vi "Microsync demo.vi"() -> ()   [LabVIEW 2023]
uses:
  4b1e20da-cac2-45f8-90a9-c1f199967da0.vi
  34aa4032-f9e1-440a-b4b5-18c951d9b119.vi
  <vilib>/Instr/_visa.llb/VISA Configure Serial Port (Instr).vi
  <vilib>/Instr/_visa.llb/VISA Flush IO Buffer Mask.ctl
panel:
  out "read buffer":string
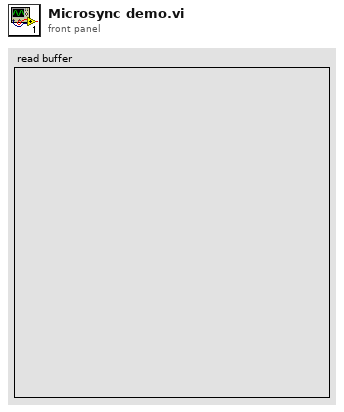
[diagram p1: front panel]
types:
  T1 = typedef "VISA Flush IO Buffer Mask.ctl" = u16
  T2 = cluster{"interval_us":u32, "N":u32, "timestamp_us":u32, "arg2":u32, "arg1":u32}
  T3 = cluster{"interval_us":u32, "N":u32, "timestamp_us":u32, "arg2":u32, "Pin":string}
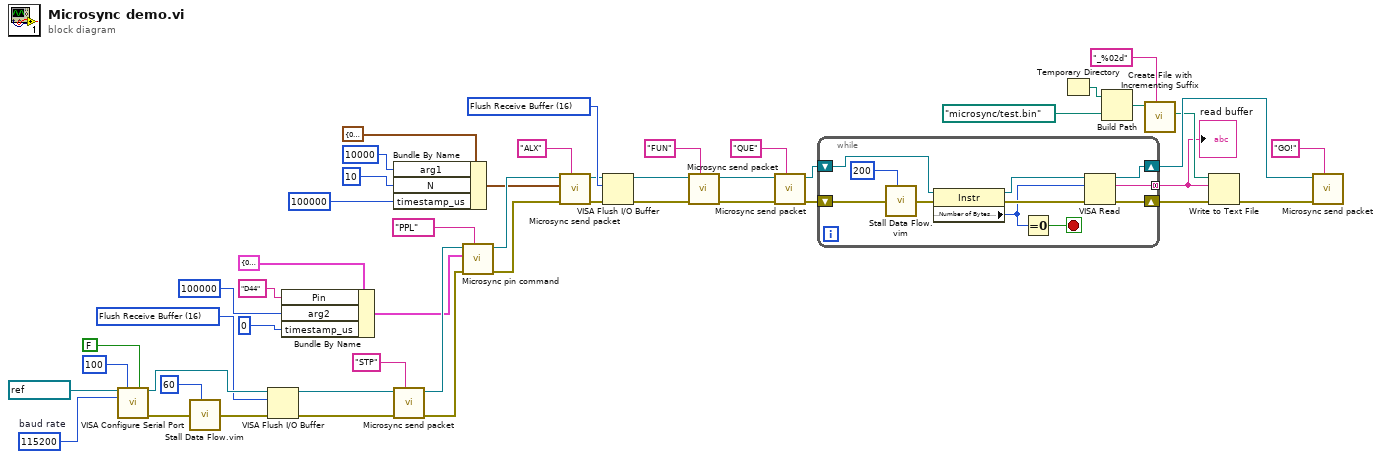
[diagram p0: block diagram]
diagram:
  w5 = T1 16 items=["Flush Receive Buffer"=16, "Write Transmit Buffer to Device"=32, "Flush Receive Buffer (No I/O)"=64, "Flush Transmit Buffer"=128] ("Mask")
  w6 = T1 16 items=["Flush Receive Buffer"=16, "Write Transmit Buffer to Device"=32, "Flush Receive Buffer (No I/O)"=64, "Flush Transmit Buffer"=128] ("Mask")
  w48 = u32 115200  # baud rate
  n1 = call-poly "VISA Configure Serial Port"("VISA resource name"=refnum<visa-resource-name> "COM5", "timeout (10sec)"=u32 100, "Enable Termination\nChar (T)"=FALSE ("Enable Termination\nChar (T)"), "baud rate (9600)"=w48) -> ("VISA resource name out"=w47:refnum<visa-resource-name>, "error out"=w46:errorcluster)  [unwired: 10 in]
  n2 = call "Stall Data Flow.vim"("value in"=w46, "milliseconds to wait"=u32 60) -> ("value out"=w45:errorcluster)  [unwired: 1 out]
  n3 = VISA Flush I/O Buffer(VISA resource name=w47, mask (16)=w6, error in (no error)=w45) -> (VISA resource name out=w34:refnum<visa-resource-name>, error out=w33:errorcluster)
  n4 = Bundle By Name(cluster=T3 {"interval_us"=0, "N"=0, "timestamp_us"=0, "arg2"=0, "Pin"=""} ("Arguments"), "Pin"="D44", "arg2"=u32 100000, "timestamp_us"=u32 0) -> (w36:T3)
  n5 = Bundle By Name(cluster=T2 {"interval_us"=0, "N"=0, "timestamp_us"=0, "arg2"=0, "arg1"=0} ("Arguments"), "arg1"=u32 10000, "N"=u32 10, "timestamp_us"=u32 100000) -> (w28:T2)
  n6 = call "Microsync send packet.vi"("Command"="STP", "error in (no error)"=w33, "VISA resource name"=w34) -> ("error out"=w35:errorcluster, "VISA resource name out"=w41:refnum<visa-resource-name>)  [unwired: 6 in, 1 out]
  n7 = call "Microsync pin command.vi"("Combo Box"="PPL", "error in (no error)"=w35, "Arguments"=w36, "VISA resource name"=w41) -> ("error out"=w24:errorcluster, "VISA resource name out"=w30:refnum<visa-resource-name>)  [unwired: 5 in, 1 out]
  n8 = call "Microsync send packet.vi"("Command"="ALX", "error in (no error)"=w24, "Arguments"=w28, "VISA resource name"=w30) -> ("error out"=w1:errorcluster, "VISA resource name out"=w4:refnum<visa-resource-name>)  [unwired: 5 in, 1 out]
  n9 = VISA Flush I/O Buffer(VISA resource name=w4, mask (16)=w5, error in (no error)=w1) -> (VISA resource name out=w3:refnum<visa-resource-name>, error out=w2:errorcluster)
  n10 = call "Microsync send packet.vi"("Command"="FUN", "error in (no error)"=w2, "VISA resource name"=w3) -> ("error out"=w13:errorcluster, "VISA resource name out"=w14:refnum<visa-resource-name>)  [unwired: 6 in, 1 out]
  n11 = call "Microsync send packet.vi"("Command"="QUE", "error in (no error)"=w13, "VISA resource name"=w14) -> ("error out"=w7:errorcluster, "VISA resource name out"=w10:refnum<visa-resource-name>)  [unwired: 6 in, 1 out]
  n12 = while {
    shift-right: [w51] -> w16
    shift-left: w7 -> [w53]
    shift-right: [w60] -> w19
    shift-left: w10 -> [w58]
    tunnel: [w59] -> w17 mode=concatenating
    stop <- w56 stop-if-true
    n13 = call "Stall Data Flow.vim"("value in"=w53, "milliseconds to wait"=u32 200) -> ("value out"=w52:errorcluster)  [unwired: 1 out]
    n14 = property class="Instr"(reference=w58, error in=w52) -> (reference out=w57:refnum<visa-resource-name>, error out=w55:errorcluster, "Serial Settings:Number of Bytes at Serial Port"=w50:u32)
    n15 = Equal To 0?(x=w50) -> (x = 0?=w56:bool)
    n16 = VISA Read(VISA resource name=w57, byte count=w50, error in (no error)=w55) -> (VISA resource name out=w60:refnum<visa-resource-name>, read buffer=w59:string, error out=w51:errorcluster)  [unwired: 1 out]
  }
  "read buffer" <- w17
  n17 = Temporary Directory() -> (w22:path)
  n18 = Build Path(base path=w22, name or relative path=path "microsync/test.bin") -> (appended path=w21:path)
  n19 = call <vilib>:"Create File with Incrementing Suffix.vi"("format string (\" (%d)\")"="_%02d" ("format string (\" (%d)\")"), "file path"=w21) -> ("actual path"=w18:path)  [unwired: 7 in, 2 out]
  n20 = Write to Text File(file (use dialog)=w18, text=w17, error in=w16) -> (error out=w15:errorcluster)  [unwired: 1 in, 2 out]
  n21 = call "Microsync send packet.vi"("Command"="GO!", "error in (no error)"=w15, "VISA resource name"=w19) -> ()  [unwired: 6 in, 3 out]
